vi "Auto Zero.vi"(8 "error in (no error)":errorcluster, 9 "Auto Zero (1: Enable)":i32(ring)=1 items=["Disable", "Enable", "Once"], 10 "Zero Type (0: Current DC)":i32(ring) items=["Current DC", "Resistance", "Temperature", "Voltage DC"], 11 "VISA resource name":refnum<visa-resource-name>) -> (0 "error out":errorcluster, 3 "VISA resource name out":refnum<visa-resource-name>)   [LabVIEW 2020, in "Agilent 3446X Series.lvlib"]
doc: "Enables or disables the auto zero mode for the specified measurements.\n\n<b>Note(s):</b>\nThis vi is not supported for EDU34450A model."
uses:
  <instrlib>/Agilent 3446X Series/Agilent 3446X Series.lvlib
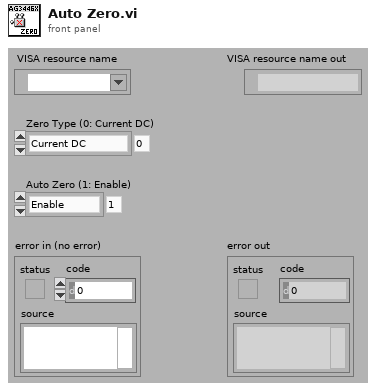
[diagram p1: front panel]
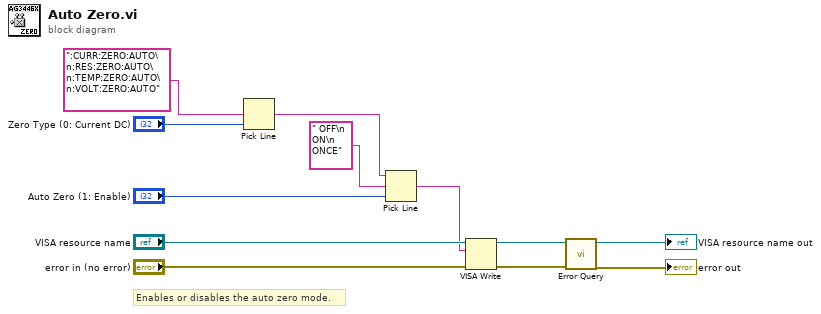
[diagram p0: block diagram]
diagram:
  # "Enables or disables the auto zero mode."
  n1 = Pick Line(multi-line string=":CURR:ZERO:AUTO\n:RES:ZERO:AUTO\n:TEMP:ZERO:AUTO\n:VOLT:ZERO:AUTO", line index="Zero Type (0: Current DC)") -> (output string=w4:string)  [unwired: 1 in]
  n2 = Pick Line(string ("")=w4, multi-line string=" OFF\n ON\n ONCE", line index="Auto Zero (1: Enable)") -> (output string=w1:string)
  n3 = VISA Write(VISA resource name="VISA resource name", write buffer=w1, error in (no error)="error in (no error)") -> (VISA resource name out=w10:refnum<visa-resource-name>, error out=w9:errorcluster)  [unwired: 1 out]
  n4 = call <instrlib>:"Error Query.vi"("error in (no error)"=w9, "VISA resource name"=w10) -> ("error out"=→"error out":errorcluster, "VISA resource name out"=→"VISA resource name out":refnum<visa-resource-name>)  [unwired: 8 out]
